vi "Filter&RemoveDuplicateErrorCodes.vi"(8 "ErrorIn":errorcluster, 10 "MainQIn":refnum<queue>, 11 "ErrorCodeIn":i32) -> (0 "ErrorOut":errorcluster, 2 "MainQOut":refnum<queue>, 3 "ErrorCodeOut":i32)   [LabVIEW 2018]
doc: "Scan through <B>QueueIn</B> and look for any queue elements that store errors. Remove any of these elements from the queue that match <B>ErrorCodeIn</B>. All other error and non-error queue elements remain on the queue and are passed to <B>QueueOut</B>. \n\nCopyright © 2016 Epimedia, Inc. All Rights Reserved.\n\nThe Epimedia Application Library is Copyright © 2009-2016 Epimedia, Inc. \nAll Rights Reserved. Used under license."
uses:
  Queue/MainQueueElements.ctl
panel:
  # "Copyright © 2016 Epimedia, Inc. All Rights Reserved.\n\nThe Epimedia Application Library is Copyright © 2009-2016 Epimedia, Inc. \nAll Rights Reserved. Used under license."
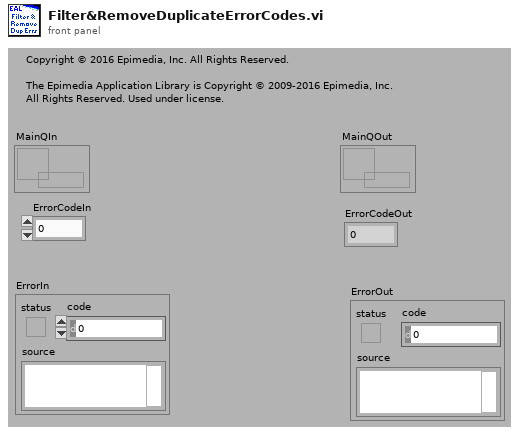
[diagram p1: front panel]
types:
  T1 = typedef "MainQueueElements.ctl" = enum16{"Spvsr_InitQ", "Spvsr_RfrshPnl", "Spvsr_InitSW", "Spvsr_InitCtrls", "Spvsr_Cursors", "Spvsr_StrtHWLp", "Spvsr_Stop", "Spvsr_NewData", "Spvsr_ScaleGraphs", "Spvsr_Error", "Spvsr_About", "Spvsr_Config", "Spvsr_FPConfig", "Spvsr_AlarmCfg", "Spvsr_DigitzOffs", "FP_AO_ctrl", "Spvsr_RestartWarn", "Spvsr_AutoCenter", "Spvsr_TrackRate", "Spvsr_ChkTime", "Spvsr_Admin", "Spvsr_Exit"}
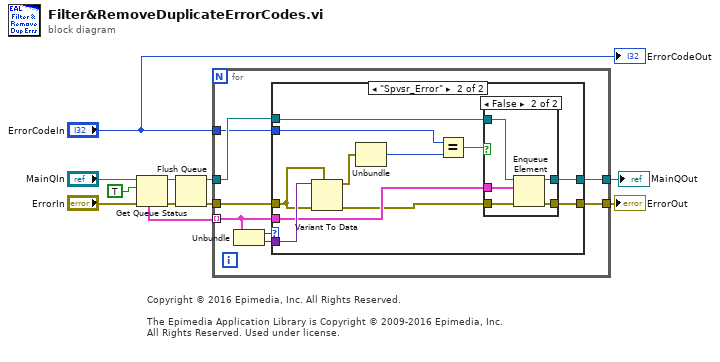
[diagram p0: block diagram]
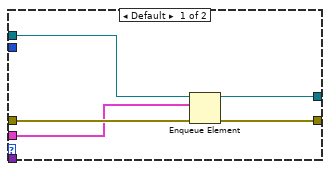
[diagram p2: hidden frame]
diagram:
  # "Copyright © 2016 Epimedia, Inc. All Rights Reserved.\n\nThe Epimedia Application Library is Copyright © 2009-2016 Epimedia, Inc. \nAll Rights Reserved. Used under license."
  n1 = Get Queue Status(queue="MainQIn", return elements? (F)=TRUE, error in (no error)="ErrorIn") -> (queue out=w8:refnum<queue>, error out=w9:errorcluster, elements=w10:cluster{"QElmnt":T1, "Data":variant}[])  [unwired: 5 out]
  n2 = Flush Queue(queue=w8, error in (no error)=w9) -> (queue out=w6:refnum<queue>, error out=w7:errorcluster)  [unwired: 1 out]
  n3 = for {
    tunnel: w10 -> [w18] mode=indexing
    tunnel: w6 -> [w15]
    tunnel: "ErrorCodeIn" -> [w14]
    tunnel: [w12] -> w1
    tunnel: w7 -> [w17]
    tunnel: [w16] -> w11
    n4 = Unbundle(w18) -> ("QElmnt"=w13:T1, "Data"=w19:variant)
    n5 = case shown="\"Spvsr_Error\"" w13 {
      tunnel: w19 -> [_ w35]
      tunnel: w18 -> [w21 w32]
      tunnel: w17 -> [w23 w26]
      tunnel: [w22 w30] -> w16
      tunnel: w15 -> [w24 w33]
      tunnel: w14 -> [_ w29]
      tunnel: [w20 w27] -> w12
      frame Default {
        n6 = Enqueue Element(queue=w24, element=w21, error in (no error)=w23) -> (queue out=w20:refnum<queue>, error out=w22:errorcluster)  [unwired: 1 in, 1 out]
      }
      frame "Spvsr_Error" {
        n7 = Variant To Data(error in=w26, type=w26, Variant=w35) -> (data=w34:errorcluster, error out=w31:errorcluster)
        n8 = Unbundle(w34) -> ("code"=w25:i32)  [unwired: 2 out]
        n9 = Equal?(x=w29, y=w25) -> (x = y?=w28:bool)
        n10 = case shown="False" w28 {
          tunnel: w33 -> [w36 w42]
          tunnel: w32 -> [_ w41]
          tunnel: w31 -> [w37 w40]
          tunnel: [w37 w39] -> w30
          tunnel: [w36 w38] -> w27
          frame True {
          }
          frame False {
            n11 = Enqueue Element(queue=w42, element=w41, error in (no error)=w40) -> (queue out=w38:refnum<queue>, error out=w39:errorcluster)  [unwired: 1 in, 1 out]
          }
        }
      }
    }
  }
  "ErrorOut" <- w11
  "MainQOut" <- w1
  "ErrorCodeOut" <- "ErrorCodeIn"
